vi "Bug2Test_TimEdit.vi"() -> ()   [LabVIEW 2013]
doc: "This example continually replans a path from Start to Goal while following the best known path, including through obstacles if necessary.\nThe Anytime D* search algorithm is useful when the world or the robot's understanding of the world is changing. Anytime D* maintains more information than the A* search algorithm so the robot can backtrack and find a new path more easily if it discovers the original path will not work."
uses:
  Bug2/Bug_StartGoalData.ctl
panel:
  in  "Loop Time":u32=100
  out "Current Y":i32
  out "Current X":i32
  in  "y Goal":i32
  in  "x Goal":i32
  in  "Random Obstacles?":bool
  in  "% Random Obstacles":dbl=40.0 min=0.0 max=100.0 step=1.0 format="%#_3g"
  out "path on obstacles":dbl[][](graph)
  in  "y start":i32
  in  "x start":i32
  # "Overview: O\nInstructions:\n1. Run the VI"
  # "Configuration"
  # "X"
  # "Y"
  # "Start"
  # "X"
  # "Y"
  # "Goal"
  # "Robot"
  # "Obstacle"
  # "Unknown"
  # "Free"
  # "Path"
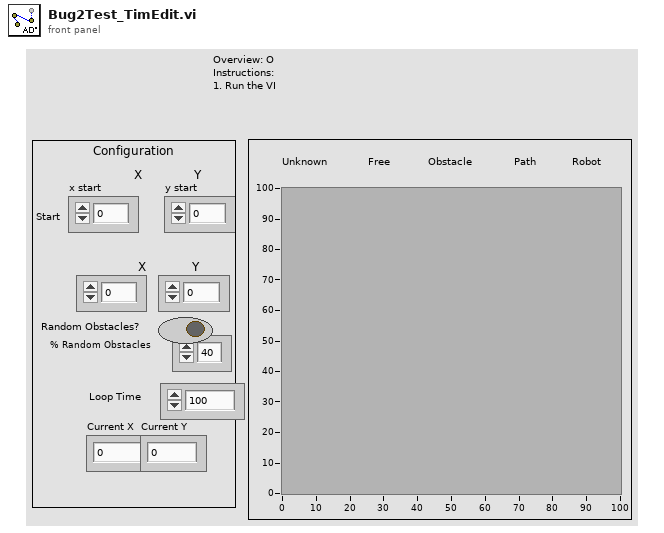
[diagram p1: front panel]
types:
  T1 = typedef "Bug_StartGoalData.ctl" = cluster{"x current":i32, "x current -1":i32, "y current":i32, "y current -1":i32, "x Goal":i32, "y Goal":i32, "x Line coords":i32[], "y Line coords":i32[], "Occ Grid":dbl[][]}
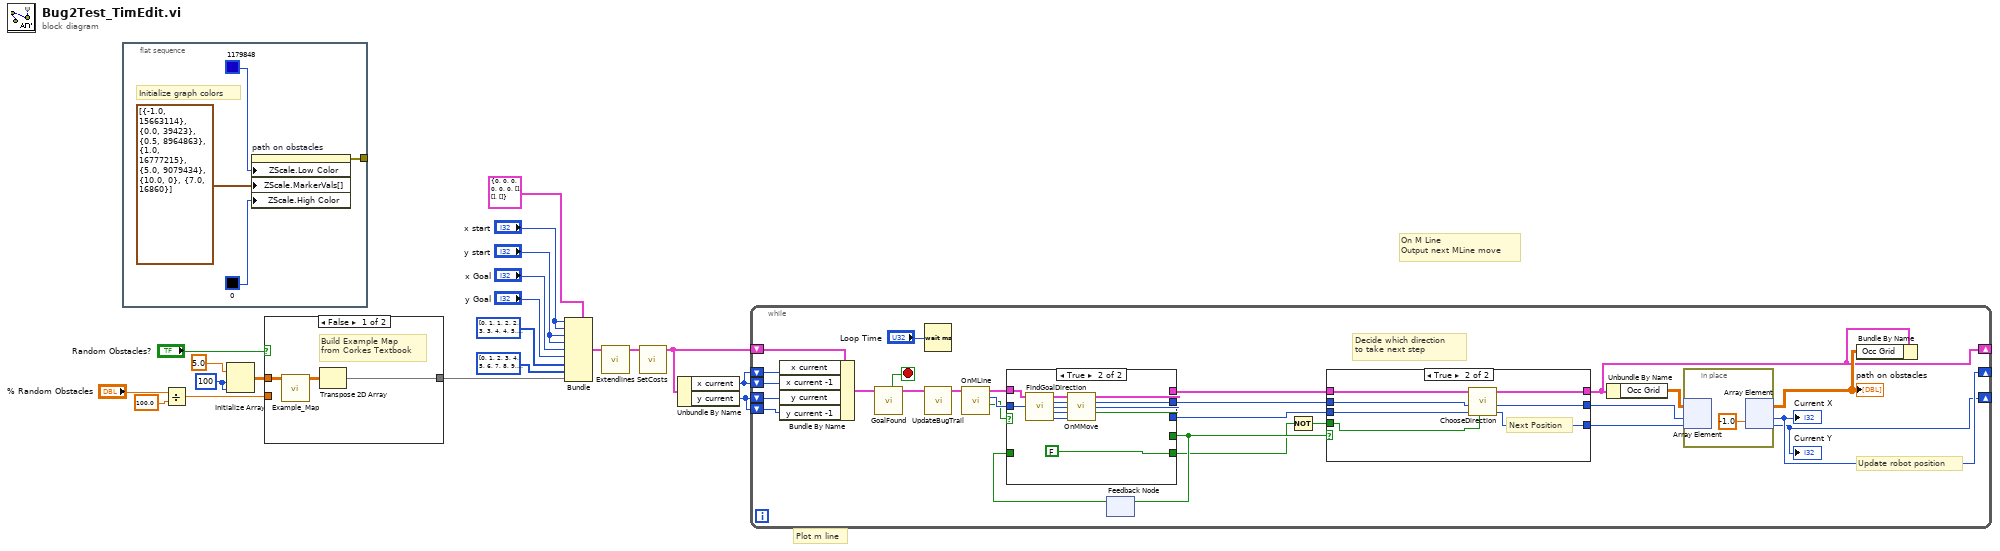
[diagram p0: block diagram]
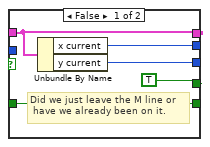
[diagram p2: hidden frame]
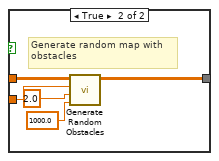
[diagram p4: hidden frame]
diagram:
  w12 = 100 ("dimension size")
  # "On M Line\nOutput next MLine move"
  # "Plot m line"
  n1 = flat-sequence {
    tunnel: [w21] -> _
    frame #0 {
      # "Initialize graph colors"
      n2 = property on="path on obstacles" class="IntGraph (strict)"("ZScale.Low Color"=u32 1179848, "ZScale.MarkerVals[]"=cluster{dbl, u32}[] [{-1.0, 15663114}, {0.0, 39423}, {0.5, 8964863}, {1.0, 16777215}, {5.0, 9079434}, {10.0, 0}, {7.0, 16860}], "ZScale.High Color"=u32 0) -> (error out=w21:errorcluster)  [unwired: 2 in, 1 out]
    }
  }
  n3 = Divide(x="% Random Obstacles", y=100.0) -> (x/y=w16:dbl)
  n4 = Initialize Array(5.0 ("\"unknown\" value for map"), w12, w12) -> (w15:dbl[][])
  n5 = case shown="False" "Random Obstacles?" {
    tunnel: w16 -> [_ w30]
    tunnel: w15 -> [w27 w29]
    tunnel: [w25 w28] -> w6
    frame False {
      # "Build Example Map\nfrom Corkes Textbook"
      n6 = call "Example_Map.vi"("Array in"=w27) -> ("Array out"=w26:dbl[][])  [unwired: 10 in]
      n7 = Transpose 2D Array(2D array=w26) -> (transposed array=w25:dbl[][])
    }
    frame True {
      # "Generate random map with\nobstacles"
      n8 = call "Generate Random Obstacles.vi"("obstacle cost"=1000.0, "free cost"=2.0, "chance"=w30, "cost in"=w29) -> ("cost out"=w28:dbl[][])  [unwired: 7 in]
    }
  }
  n9 = Bundle(cluster=T1 {"x current"=0, "x current -1"=0, "y current"=0, "y current -1"=0, "x Goal"=0, "y Goal"=0, "x Line coords"=[], "y Line coords"=[], "Occ Grid"=[]} ("Start Goal Data"), "x current"="x start", "x current -1"="x start", "y current"="y start", "y current -1"="y start", "x Goal"="x Goal", "y Goal"="y Goal", "x Line coords"=i32[] [0, 1, 1, 2, 2, 3, 3, 4, 4, 5, 5, 6, 6, 7, 7, 8, 8, 9, 9, 10, 10, 11, 11, 12, 12, 13, 13, 14, 14, 15, 15, 16, 16, 17, 17, 18, 18, 19, 19, 20, 20, 21, 21, 22, 22, 23, 23, 24, 24, 25, 25, 26, 26, 27, 27, 28, 28, 29, 29, 30, 30, 31, 31, 32, 32, 33, 33, 34, 34, 35, 35, 36, 36, 37, 37, 38, 38, 39, 39, 40, 40, 41, 41, 42, 42, 43, 43, 44, 44, 45, 45, 46, 46, 47, 47, 48, 48, 49, 49, 50, 50], "y Line coords"=i32[] [0, 1, 2, 3, 4, 5, 6, 7, 8, 9, 10, 11, 12, 13, 14, 15, 16, 17, 18, 19, 20, 21, 22, 23, 24, 25, 26, 27, 28, 29, 30, 31, 32, 33, 34, 35, 36, 37, 38, 39, 40, 41, 42, 43, 44, 45, 46, 47, 48, 49, 50, 51, 52, 53, 54, 55, 56, 57, 58, 59, 60, 61, 62, 63, 64, 65, 66, 67, 68, 69, 70, 71, 72, 73, 74, 75, 76, 77, 78, 79, 80, 81, 82, 83, 84, 85, 86, 87, 88, 89, 90, 91, 92, 93, 94, 95, 96, 97, 98, 99, 100], "Occ Grid"=w6) -> (w5:T1)
  n10 = call "Extendlines.vi"("Start Goal Data"=w5) -> ("Start Goal Data out"=w11:T1)  [unwired: 10 in]
  n11 = call "SetCosts.vi"("Start Goal Data"=w11) -> ("Start Goal Data out"=w3:T1)  [unwired: 10 in]
  n12 = Unbundle By Name(w3) -> ("x current"=w13:i32, "y current"=w14:i32)
  n13 = while {
    shift-right: [w51] -> _
    shift-left: w13 -> [w44]
    shift-right: [w50] -> _
    shift-left: w14 -> [w42]
    shift-left: w13 -> [w43]
    shift-left: w14 -> [w41]
    shift-right: [w36] -> _
    shift-left: w3 -> [w45]
    stop <- w49 stop-if-true
    # "Decide which direction \nto take next step"
    # "Update robot position"
    n14 = Bundle By Name(cluster=w45, "x current"=w44, "x current -1"=w43, "y current"=w42, "y current -1"=w41) -> (w40:T1)
    n15 = call "GoalFound.vi"("Start Goal Data"=w40) -> ("Start Goal Data out"=w39:T1, "Boolean"=w49:bool)  [unwired: 9 in]
    n16 = Wait (ms)(milliseconds to wait="Loop Time") -> ()  [unwired: 1 out]
    n17 = call "UpdateBugTrail.vi"("Start Goal Data"=w39) -> ("Start Goal Data out"=w48:T1)  [unwired: 10 in]
    n18 = call "OnMLine.vi"("Start Goal Data"=w48) -> ("On the Line?"=w33:bool, "Match Index"=w34:i32, "Start Goal Data out"=w47:T1)  [unwired: 8 in]
    n19 = feedback #1() -> (w55:bool)  [unwired: 1 in]
    n20 = case shown="True" w33 {
      tunnel: [TRUE w77] -> w56
      tunnel: [w64 w72] -> w59
      tunnel: [w63 w71] -> w58
      tunnel: w34 -> [_ w68]
      tunnel: w55 -> [w61 _]
      tunnel: [w61 FALSE] -> w54
      tunnel: w47 -> [w62 w67]
      tunnel: [w62 w70] -> w46
      frame False {
        # "Did we just leave the M line or\n have we already been on it."
        n21 = Unbundle By Name(w62) -> ("x current"=w64:i32, "y current"=w63:i32)
      }
      frame True {
        n22 = call "FindGoalDirection.vi"("Start Goal Data in"=w67, "Match Index"=w68) -> ("Start Goal Data out"=w66:T1, "x1 4"=w76:i32, "x1 3"=w75:i32, "x1 2"=w74:i32, "x1"=w73:i32)  [unwired: 9 in]
        n23 = call "OnMMove.vi"("Start Goal Data"=w66, "x1 4"=w76, "x1 3"=w75, "x1 2"=w74, "x1"=w73) -> ("Start Goal Data out"=w70:T1, "x out"=w72:i32, "y out"=w71:i32, "Boolean"=w77:bool)  [unwired: 5 in, 2 out]
      }
    }
    n24 = feedback-in #1(w56) -> ()
    n25 = Not(x=w54) -> (.not. x?=w35:bool)
    n26 = case shown="True" w56 {
      tunnel: w59 -> [w79 w87]
      tunnel: w58 -> [w80 w85]
      tunnel: [w79 w82] -> w53
      tunnel: [w80 w83] -> w52
      tunnel: w35 -> [_ w86]
      tunnel: w46 -> [w78 w84]
      tunnel: [w78 w81] -> w36
      frame False {
      }
      frame True {
        # "Next Position"
        n27 = call "ChooseDirection.vi"("Boolean"=w86, "y in"=w85, "x in"=w87, "Start Goal Data"=w84) -> ("y out"=w83:i32, "x out 2"=w82:i32, "Start Goal Data out"=w81:T1)  [unwired: 5 in]
      }
    }
    n28 = Unbundle By Name(w36) -> ("Occ Grid"=w38:dbl[][])
    n29 = in-place {
      n30 = in-place-array #2(w38, w53, w52) -> ()  [unwired: 1 out]
      n31 = in-place-array #2(-1.0) -> (w37:dbl[][], w51:i32, w50:i32)
    }
    "path on obstacles" <- w37
    "Current X" <- w51
    "Current Y" <- w50
    n32 = Bundle By Name(cluster=w36, "Occ Grid"=w37) -> ()  [unwired: 1 out]
  }
